vi "LauncherGui.vi"() -> ()   [LabVIEW 2016]
uses:
  LauncherGui.Action.ctl
  Drivers/FestoCPX/FestoCPX.State.ctl
  Drivers/V7310/V7310.Data.Status.State.ctl
  Drivers/KeyenceCVX/public/KeyenceCVX.Data.Status.State.ctl
  Drivers/Keyence/Keyence.Data.Status.State.ctl
  tools/Translator/Translator.Message.ctl
  tools/Translator/Translator.FormatMessage.vi
  Database/Database.Global.vi
  Drivers/FestoCPX/FestoCPX.Global.vi
  Drivers/V7310/LowLevel/V7310.Global.vi
  Drivers/Keyence/LowLevel/Keyence.Global.vi
  Global/ApplicationGlobal.vi
  tools/Translator/Translator.Global.vi
panel:
  out "FestoCPX":bool caption="Festo CPX"
  out "OrderScanner":bool caption="Skaner Zlecenia"
  out "ProdScanner":bool caption="Skaner Produktu"
  out "Laser":bool caption="Laser Videojet"
  out "Header":string
  out "_loop":i32(ring)=4
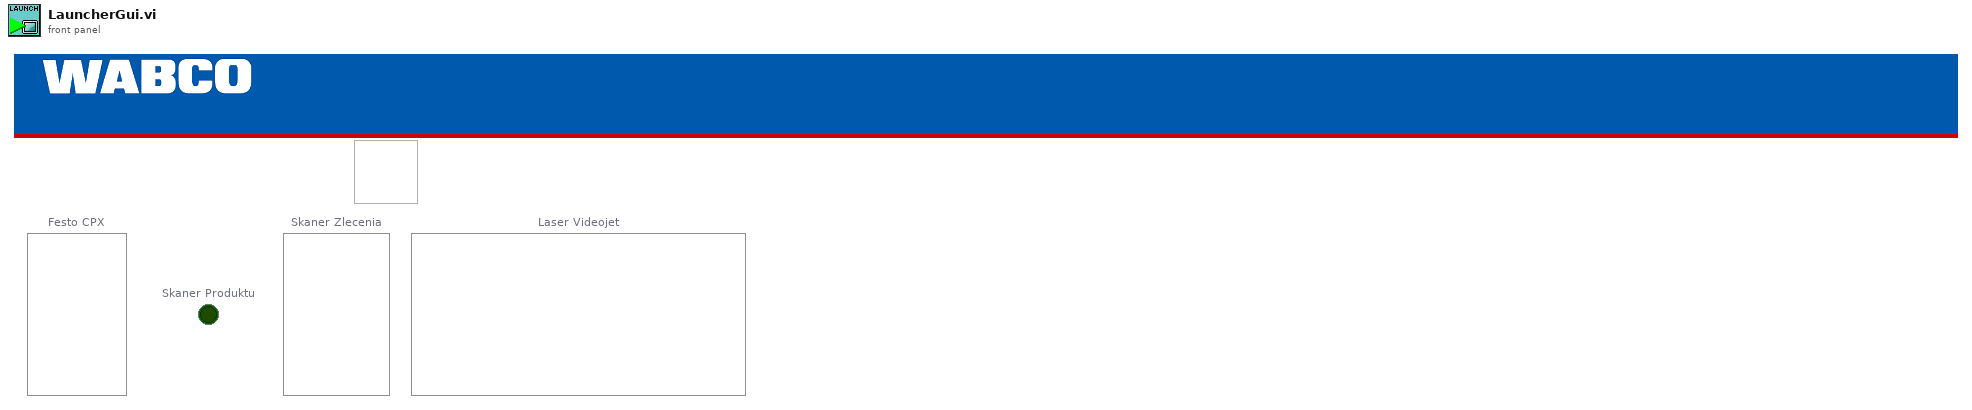
[diagram p1: front panel]
types:
  T1 = typedef "LauncherGui.Action.ctl" = enum32{"idle", "constructor", "destructor", "--- LauncherGui ---"}
  T2 = typedef "FestoCPX.State.ctl" = enum16{"First", "Error", "Init", "Run"}
  T3 = typedef "V7310.Data.Status.State.ctl" = enum16{"First", "Init", "Msg", "Error", "Abort", "Idle", "Run"}
  T4 = typedef "KeyenceCVX.Data.Status.State.ctl" = enum16{"Init", "Idle", "Scan", "Reset", "ScanAck", "ChangeProgram"}
  T5 = typedef "Keyence.Data.Status.State.ctl" = enum16{"First", "Init", "Reset", "Idle", "Scan", "Tune"}
  T6 = typedef "Translator.Message.ctl" = enum16{"-", "Event confirmed", "Log out", "Log in", "Shutdown", "Cancel", "Start", "Begin time", "End time", "Duration", "Service Mode", "Ignore Results", "Serial Format", "On", "Off", "OK", "NOK", "NOK %s", "Home", "Work", "Close", "Open", "In progress...", "Missing", "Empty", "Hardware failure", "Initial", "Default", "Total", "Out of range", "Free disk space is below 1GB - contact technician", "Error %d >> %s", "Error %d >> %s >> %s", "Msg %d >> %s", "Laser msg %d %s", "Laser cmd error %s %d", "Laser cmd failed %s", "Laser cmd warning %s", "Laser disconnected", "Laser status %s", "Laser already started", "Laser job unkonwn %s", "Laser job missing %s", "Laser job select failure %s", "Unable to start laser printing (%s)", "Unable to stop laser printing (%s)", "Laser marking aborted", "Laser marking timeout", "Unable to reset Laser Interlock (%s)", "Unable to trigger Laser. Laser not ready (%s)", "Laser job '%s' coordinates not configured", "Starting %s", "Quitting %s", "Configured", "Initializing", "Quitting", "Loading", "Loaded %d results", "Loaded %d events", "Running", "Stopped", "Summary", "Laser", "Do you want to continue?", "Do you want to delete the configuration?", "The configuration is being used by an order. Unable to delete!", "Press confirm button", "Station is not based. Do you want to exit?", "Station requires changeover. Do you want to run the test?", "Test options are not set as default. Do you want to continue?", "Formatting of WabcoNo is disabled. Do you want to continue?", "Product not detected. Do you want to continue?", "Product scan failed. Do you want to continue?", "Calibration", "Log out?", "System", "All", "IDLE", "Translating...%s", "Not found", "Alarm %s", "Run", "Skip", "Abort", "Repeat", "Please wait...", "Database disconnected", "Database disconnected - changeover disabled!", "Login to database successful", "Login to database failed: %d; %s", "Unable to check the product status of reference %d - database disconnected", "Unable to set the product status of reference %d - database disconnected", "Variant file backup %s", "Read variant (%s)", "Result", "Station armed!", "Station requires changeover!", "Select reference number...", "EMERGENCY BUTTON - press Control button", "EMERGENCY DOOR - press Control button", "Resetting Emergency...", "Unable to reset safety circuit - Emergency Button pressed", "Unable to reset safety circuit - Emergency Side Door open", "Station not based", "Station based", "Station not empty", "Station basing...", "No order", "Press Start to begin new order", "Scanning new order", "Order NOK. Correct or scan again", "Order OK. Press Accept", "Order ready", "Revolver incorrect", "Fork incorrect", "Revolver missing", "Revolver empty", "Container missing", "Offline results", "Offline statistics", "Updating statistics %.1f %%", "DMC Configurator", "Door open", "Close the front door", "Press start button", "Done. Open the front door", "Running...", "Running...%.1f %%", "Pause %s", "Pause %s. NOK container missing", "Pause %s. OK container missing", "Pause %s. Revolver empty", "Pause %s. Revolver missing", "Pause %s. Revolver incorrect", "Pause %s. Fork missing", "Pause %s. Fork incorrect", "Pause %s. Too many failures", "Pause %s. Unloading failure", "Pause %s. One slot is not working", "Pause %s. Part order is done. Empty OK container", "Pause %s. Unable to move product to slot", "Pause %s. Unable to move back product pusher", "Pause %s. Unable to lift product", "Pause %s. Unable to move back product lifter", "Pause %s. Unable to move product arm to Work", "Pause %s. Unable to move product arm to NOK", "Pause %s. Unable to move product arm to OK", "Pause %s. Unable to unsuck the NOK product", "Pause %s. Unable to drop the NOK product", "Pause %s. Product OK missing", "Pause %s. Unable to unsuck the OK product", "Pause %s. Unable to drop the OK product", "Stopping...", "File '%s' is missing", "File '%s' is broken", "File '%s' is running", "Log file started (%s)", "Log file ended (%s)", "Log file stopped (%s)", "Log file ignored (%s)", "Log file exported (%s)", "Log file export failed (%s)", "Wrong serial number in log file", "Wrong reference number in log file", "Test steps are missing", "%s = %.3f", "Process param '%s' not found in DB", "Process param '%s' wrong order", "Process param '%s' value %.3f out of limits (%.3f; %.3f)", "Step%d param '%s' not found in DB", "Step%d param '%s' wrong order", "Step%d param '%s' value %.3f out of limits (%.3f; %.3f)", "Step%d EV '%s' not found in DB", "Step%d EV '%s' wrong order", "\"%s\" not found in DB", "\"%s\" wrong order", "\"%s\" value %.3f out of limits (%.3f; %.3f)", "\"%s\" not found in software", "Process init (%s)", "Process started", "Process restarted", "Process run", "Process done", "Process done - remove OK container", "Process aborted", "Process aborted at work", "Process aborted at home", "Process error", "Process error at home", "Process error at work", "Process close", "Process pause", "Process continue", "Process door open", "Process door close", "Process pause at slot %s due to %s", "Select plate from the order to process", "Do you want to start the process?", "Do you want to continue the process?", "There is unfinished order. Do you want to put the new order?", "Product %s %d OK", "Product %s %d NOK", "Unable to unload the slot %s. Product missing in the slot", "Unable to unload the slot %s. Product already in the arm", "Unable to accept the product as OK. Product missing in slot %s", "Unable to accept the product as OK. Product could not drop into the container at slot %s", "Unable to accept the product as NOK. Product could not drop into the container at slot %s", "Scan failed. Error %s", "Scan failed. Scanner disconnected", "Scan failed. Wrong Wabco number %d, limit (%d,%d)", "Scan failed. Wrong serial number %d, limit (%d,%d)", "Scan failed. Wrong date %d, limit (%d,%d)", "Scan failed. Wrong product wabco number %d (expected %d)", "Scan failed. Wrong product serial number %d (expected > 0)", "Scan OK %s", "Scan failed. Unable to determine table position (%s)", "Scan failed. Timeout", "Tune failed. Scanner disconnected", "Tune failed. Timeout", "%s = %d", "%s = %d->%d", "Unable to set %s = %.2f - Air Pressure Inside off", "Unable to set digital output '%s' = %d", "Unable to activate air pressure inside - timeout", "Unable to activate air pressure inside - aborted", "Unable to switch on Air Main Valve - Air Pressure Inlet off", "Unable to switch on Air Main Valve - Door open", "Unable to switch off Air Main Valve - timeout", "Unable to switch off Air Main Valve - aborted", "Unable to rotate Table - timeout", "Unable to rotate Table - aborted", "Unable to rotate Table - Product Move not in Home position", "Unable to rotate Table - Air Pressure Inside off", "Unable to rotate Table - Product Lift A not in Home position", "Unable to rotate Table - Product Lift B not in Home position", "Unable to rotate Table - unlock before movement timeout", "Unable to rotate Table - lock after movement timeout", "Unable to move Table Lock to %s position - timeout", "Unable to move Table Lock to %s position - aborted", "Unable to move Table Lock to %s position - Air Pressure Inside off", "Unable to move Table Lock to %s position - Table not in position", "Unable to move Product Lift A to %s position - timeout", "Unable to move Product Lift B to %s position - timeout", "Unable to move Product Lift A to %s position - aborted", "Unable to move Product Lift B to %s position - aborted", "Unable to move Product Lift A to %s position - Air Pressure Inside off", "Unable to move Product Lift B to %s position - Air Pressure Inside off", "Unable to move Product Lift A to %s position - Table not locked", "Unable to move Product Lift B to %s position - Table not locked", "Unable to move Product Lift A to %s position - Product Arm not in Work position", "Unable to move Product Lift B to %s position - Product Arm not in Work position", "Unable to set Product Suction Gripper %s to %s - timeout", "Unable to set Product Suction Gripper %s to %s - aborted", "Unable to set Product Suction Gripper %s to %s - Air Pressure Inside off", "Unable to set Product Suction Gripper %s to %s - Table slot unkown", "Unable to move Product Arm to %s position - timeout", "Unable to move Product Arm to %s position - aborted", "Unable to move Product Arm to %s position - Air Pressure Inside off", "Unable to move Product Arm to %s position - Product Lift A not in Home position", "Unable to move Product Arm to %s position - Product Lift B not in Home position", "Unable to move Product to %s position - timeout", "Unable to move Product to %s position - aborted", "Unable to move Product to %s position - Air Pressure Inside off", "Unable to move Product to %s position - Table not in position"}
  T7 = enum32{"Invalid", "Default", "Floating", "Floating/Auto-Hide", "Modal"}
  T8 = typedef "Database.Main.Data.Status.ctl" = cluster{"Run":bool, "Handle":i32, "ConnTS":timestamp, "DbTime":timestamp, "DbTimeCode":dbl, "DbTimeOffset":dbl}
  T9 = typedef "FestoCPX.Data.Status.ctl" = cluster{"State":T2, "Conn":refnum<k5>, "TS":timestamp}
  T10 = typedef "V7310.Data.Status.ctl" = cluster{"State":T3, "LaserStatus":T11, "LaserStatusRaw":string, "Ref":refnum<k5>, "RTC TS":timestamp, "Conn TS":timestamp, "Msg":T12[], "JobInUse":string, "Jobs":string[], "Vars":T13[]}
  T11 = typedef "V7310.LaserStatus.ctl" = enum16{"-", "FatalError", "Initialize", "KeySwitchOpen", "TimeoutInterlock", "InterlockOpen", "StartUp", "ShutterlockOpen", "Standby", "Ready", "PrepareForMarking", "WaitForTrigger", "Marking"}
  T12 = typedef "V7310.Message.Data.ctl" = cluster{"ID":i32, "Msg":string}
  T13 = typedef "V7310.Job.Variable.ctl" = cluster{"Name":string, "Value":string}
  T14 = typedef "KeyenceCVX.Data.Status.ctl" = cluster{"State":T4, "Ref":refnum<k5>, "ProgramNo":u16, "SDCard":u8, "EndTS":timestamp, "ImgPathA":path, "ImgPathB":path, "TriggerNo":T15, "RunMode":T16}
  T15 = typedef "TriggerNo.ctl" = u8
  T16 = typedef "RunMode.ctl" = enum16{"SETUP", "RUN"}
  T17 = typedef "Keyence.Data.Status.ctl" = cluster{"State":T5, "Ref":refnum<k5>, "Bank":u8, "Version":string, "Model":string, "EndTS":timestamp, "ImgPath":path, "Tuned":bool}
  T18 = typedef "LVPositionTypeDef.ctl" = cluster{"Left":i32, "Top":i32}
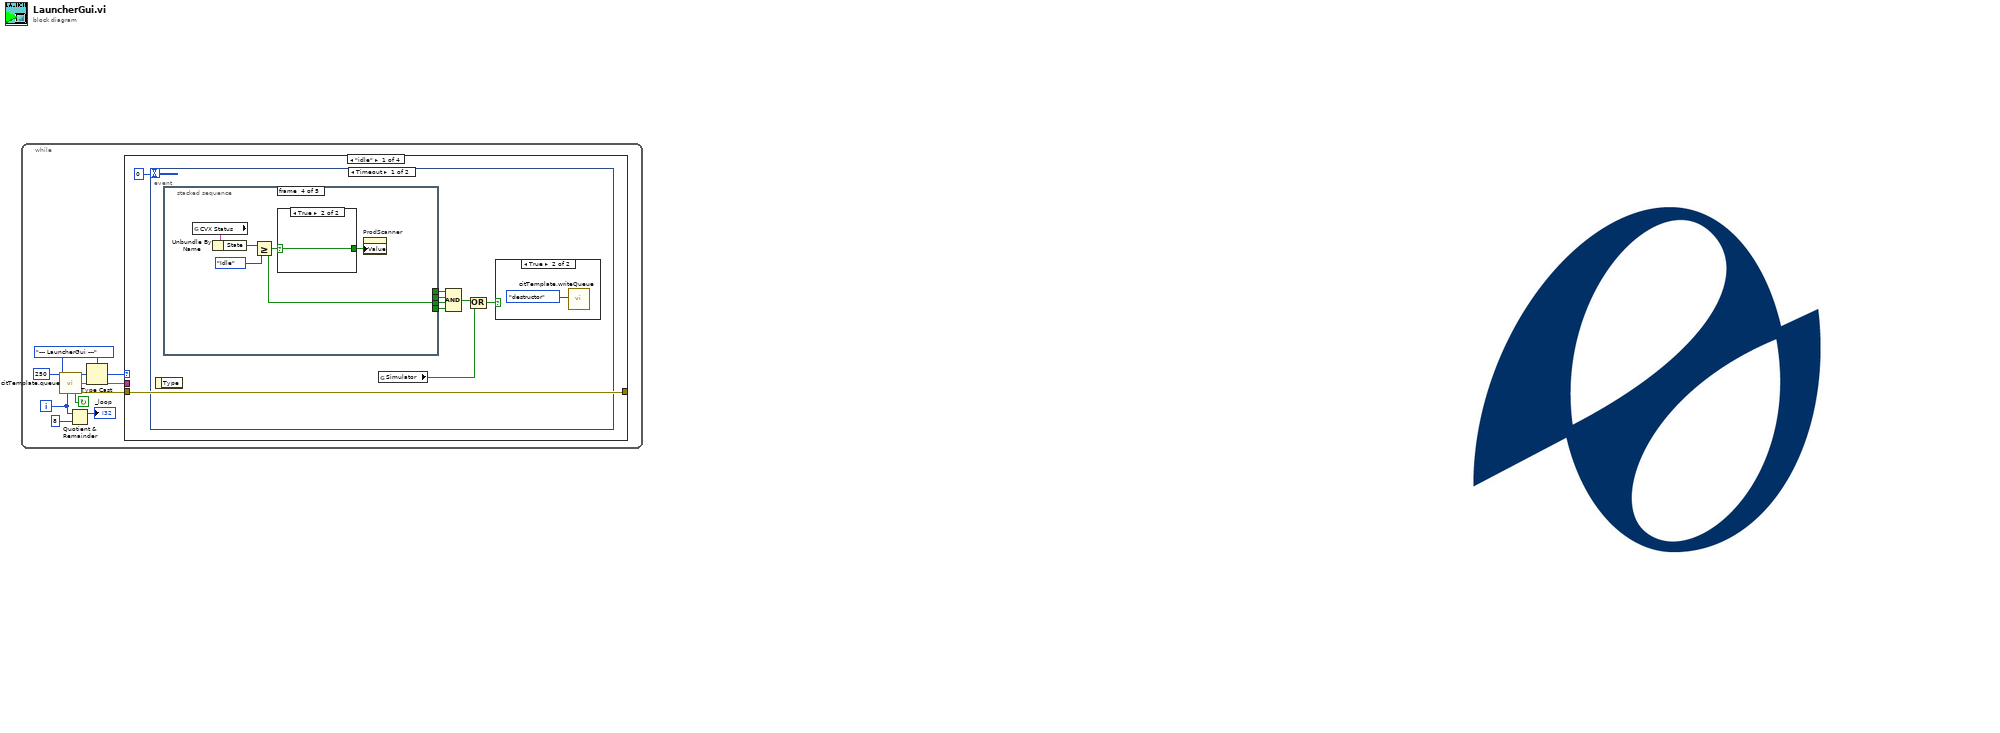
[diagram p0: block diagram]
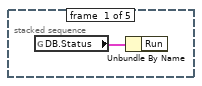
[diagram p3: hidden frame]
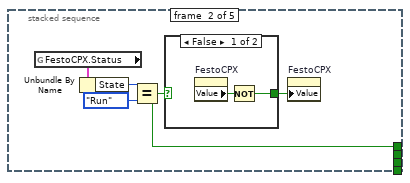
[diagram p4: hidden frame]
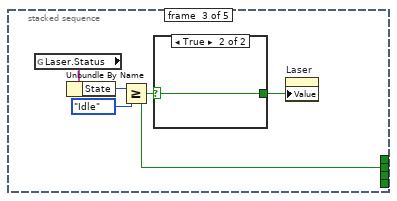
[diagram p6: hidden frame]
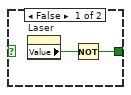
[diagram p7: hidden frame]
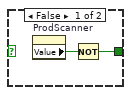
[diagram p8: hidden frame]
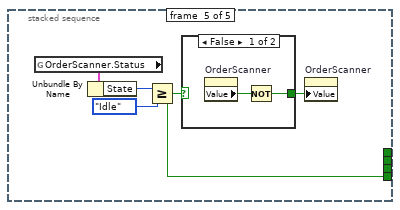
[diagram p9: hidden frame]
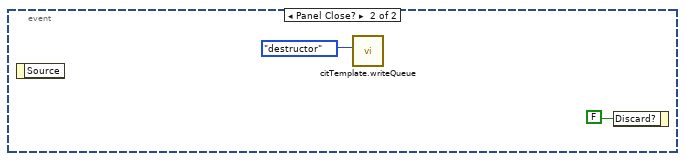
[diagram p11: hidden frame]
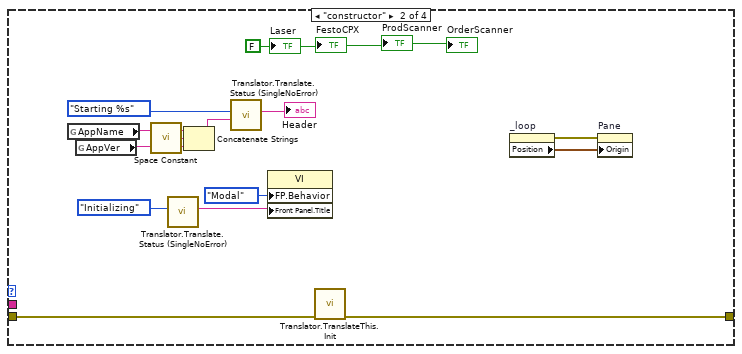
[diagram p12: hidden frame]
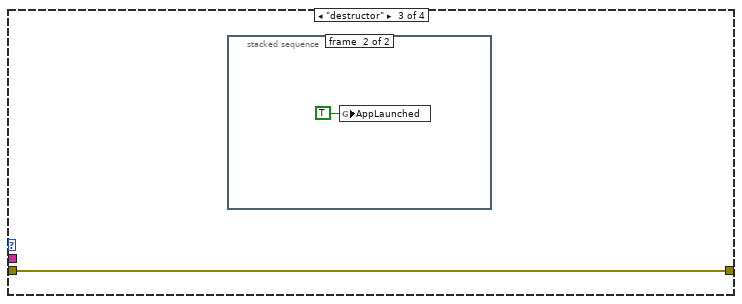
[diagram p13: hidden frame]
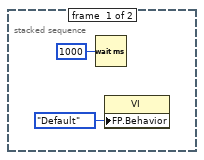
[diagram p14: hidden frame]
diagram:
  n1 = while {
    i -> [w2]
    stop <- w4 continue-if-true
    w5 = LauncherGui.Action."--- LauncherGui ---" ("Action")
    n2 = call "citTemplate.queue.vi"("ms timeout (250 ms)"=250, "event enum"=w5, "iteration (-1)"=w2) -> ("event out"=w9:u32, "(flatten) data out"=w6:string, "continue"=w4:bool, "error out"=w7:errorcluster)  [unwired: 2 in, 7 out]
    n3 = Quotient & Remainder(x=w2, y=8) -> (x-y*floor(x/y)=→"_loop":i32)  [unwired: 1 out]
    n4 = Type Cast(type=w5, x=w9) -> (*(type *) &x=w8:T1)
    n5 = case shown="\"idle\"" w8 {
      tunnel: w7 -> [w11 w59 w70 w74]
      tunnel: w6 -> [_ _ _ _]
      tunnel: [w11 w58 w70 w74] -> _
      frame "idle" {
        n6 = event shown="[0] Timeout" {
          selector: _ -> [_ _]
          dyn-events: _ -> [_ _]
          timeout: 0 -> [_ _]
          event Timeout {
            n7 = event-data() -> ()  [unwired: 1 in, 1 out]
            n8 = stacked-sequence {
              tunnel: [_ _ w30 _ _] -> w19
              tunnel: [_ w22 _ _ _] -> w17
              tunnel: [_ _ _ w39 _] -> w16
              tunnel: [_ _ _ _ w46] -> w15
              frame #0 {
                n9 = global read "Database.Global.vi" "DB.Status"() -> (w21:T8)
                n10 = Unbundle By Name(w21) -> ()  [unwired: 1 out]
              }
              frame #1 {
                n11 = global read "FestoCPX.Global.vi" "FestoCPX.Status"() -> (w23:T9)
                n12 = Unbundle By Name(w23) -> ("State"=w24:T2)
                n13 = Equal?(x=w24, y=FestoCPX.State."Run") -> (x = y?=w22:bool)
                n14 = case shown="False" w22 {
                  selector: w22 -> [_ w29]
                  tunnel: [w28 w29] -> w26
                  frame False {
                    n15 = property on="FestoCPX" class="Bool (strict)"() -> ("Value"=w27:bool)  [unwired: 2 in, 2 out]
                    n16 = Not(x=w27) -> (.not. x?=w28:bool)
                  }
                  frame True {
                  }
                }
                n17 = property on="FestoCPX" class="Bool (strict)"("Value"=w26) -> ()  [unwired: 2 in, 2 out]
              }
              frame #2 {
                n18 = global read "V7310.Global.vi" "Laser.Status"() -> (w33:T10)
                n19 = Unbundle By Name(w33) -> ("State"=w34:T3)
                n20 = Greater Or Equal?(x=w34, y=V7310.Data.Status.State."Idle") -> (x >= y?=w30:bool)
                n21 = case shown="True" w30 {
                  selector: w30 -> [_ w37]
                  tunnel: [w36 w37] -> w31
                  frame False {
                    n22 = property on="Laser" class="Bool (strict)"() -> ("Value"=w35:bool)  [unwired: 2 in, 2 out]
                    n23 = Not(x=w35) -> (.not. x?=w36:bool)
                  }
                  frame True {
                  }
                }
                n24 = property on="Laser" class="Bool (strict)"("Value"=w31) -> ()  [unwired: 2 in, 2 out]
              }
              frame #3 {
                n25 = global read "Keyence.Global.vi" "CVX Status"() -> (w41:T14)
                n26 = Unbundle By Name(w41) -> ("State"=w42:T4)
                n27 = Greater Or Equal?(x=w42, y=KeyenceCVX.Data.Status.State."Idle") -> (x >= y?=w39:bool)
                n28 = case shown="True" w39 {
                  selector: w39 -> [_ w45]
                  tunnel: [w44 w45] -> w40
                  frame False {
                    n29 = property on="ProdScanner" class="Bool (strict)"() -> ("Value"=w43:bool)  [unwired: 2 in, 2 out]
                    n30 = Not(x=w43) -> (.not. x?=w44:bool)
                  }
                  frame True {
                  }
                }
                n31 = property on="ProdScanner" class="Bool (strict)"("Value"=w40) -> ()  [unwired: 2 in, 2 out]
              }
              frame #4 {
                n32 = global read "Keyence.Global.vi" "OrderScanner.Status"() -> (w48:T17)
                n33 = Unbundle By Name(w48) -> ("State"=w50:T5)
                n34 = Greater Or Equal?(x=w50, y=Keyence.Data.Status.State."Idle") -> (x >= y?=w46:bool)
                n35 = case shown="False" w46 {
                  selector: w46 -> [_ w53]
                  tunnel: [w52 w53] -> w47
                  frame False {
                    n36 = property on="OrderScanner" class="Bool (strict)"() -> ("Value"=w51:bool)  [unwired: 2 in, 2 out]
                    n37 = Not(x=w51) -> (.not. x?=w52:bool)
                  }
                  frame True {
                  }
                }
                n38 = property on="OrderScanner" class="Bool (strict)"("Value"=w47) -> ()  [unwired: 2 in, 2 out]
              }
            }
            n39 = global read "ApplicationGlobal.vi" "Simulator"() -> (w13:bool)
            n40 = Compound Arithmetic op=AND(w17, w19, w16, w15) -> (w18:bool)
            n41 = Compound Arithmetic op=OR(w18, w13) -> (w14:bool)
            n42 = case shown="True" w14 {
              frame False {
              }
              frame True {
                n43 = call "citTemplate.writeQueue.vi"("event in (if not connected:all statemachine with data event)"=LauncherGui.Action."destructor" ("Action")) -> ()  [unwired: 14 in, 1 out]
              }
            }
          }
          event Panel Close? {
            n44 = event-data() -> ()  [unwired: 1 in, 1 out]
            n45 = call "citTemplate.writeQueue.vi"("event in (if not connected:all statemachine with data event)"=LauncherGui.Action."destructor" ("Action")) -> ()  [unwired: 14 in, 1 out]
            n46 = event-data("Discard?"=FALSE) -> ()  [unwired: 1 in, 1 out]
          }
        }
      }
      frame "constructor" {
        w65 = FALSE ("Laser")
        n47 = global read "ApplicationGlobal.vi" "AppName"() -> (w64:string)
        n48 = global read "ApplicationGlobal.vi" "AppVer"() -> (w63:string)
        n49 = call <vilib>:"Space Constant.vi"() -> ("String"=w61:string)
        n50 = call "Translator.Translate.Status (SingleNoError).vi"("msg"=Translator.Message."Initializing") -> ("Translated Msg"=w56:string)  [unwired: 10 in]
        n51 = Concatenate Strings(w64, w61, w63) -> (w62:string)
        n52 = call "Translator.Translate.Status (SingleNoError).vi"("Argument"=w62, "msg"=Translator.Message."Starting %s") -> ("Translated Msg"=→"Header":string)  [unwired: 9 in]
        n53 = property class="VI"("FP.Behavior"=T7."Modal" ("Front Panel Window:Behavior"), "Front Panel.Title"=w56) -> ()  [unwired: 2 in, 2 out]
        n54 = call "Translator.TranslateThis.Init.vi"("error in"=w59) -> ("error out"=w58:errorcluster)  [unwired: 10 in]
        n55 = property on="_loop" class="Ring (strict)"() -> (error out=w68:errorcluster, "Position"=w69:T18)  [unwired: 2 in, 1 out]
        n56 = property on="Pane" class="Pane"(error in=w68, "Origin"=w69) -> ()  [unwired: 1 in, 2 out]
        "Laser" <- w65
        "ProdScanner" <- w65
        "OrderScanner" <- w65
        "FestoCPX" <- w65
      }
      frame "destructor" {
        n57 = stacked-sequence {
          frame #0 {
            n58 = Wait (ms)(milliseconds to wait=u32 1000) -> ()  [unwired: 1 out]
            n59 = property class="VI"("FP.Behavior"=T7."Default" ("Front Panel Window:Behavior")) -> ()  [unwired: 2 in, 2 out]
          }
          frame #1 {
            n60 = global write "ApplicationGlobal.vi" "AppLaunched"(TRUE ("AppLaunched")) -> ()
          }
        }
      }
      frame "--- LauncherGui ---" {
      }
    }
  }
